vi "example_microFPGA.vi"() -> ()   [LabVIEW 2018]
panel:
  in  "write or read 2":u16(ring)=1 items=["read", "write"]
  out "Camera_sw_start_READ":u16(ring)=1 items=["Stop = 0", "Start = 1 "]
  in  "milliseconds to RUN":u32=2000
  out "value write confirm 11":bool=TRUE
  in  "Camera_sw_start_WRITE":u16(ring)=1 items=["Stop = 0", "Start = 1 "]
  out "camera_laser_delay_time_READ":u32(slide)=500 max=65535 step=1 scale=0.0..665535.0 scale format="%u us"
  out "value write confirm 10":bool=TRUE
  in  "camera_laser_delay_time_WRITE":u32(slide)=500 max=65535 step=1 scale=0.0..65535.0 scale format="%u us"
  out "camera_exposure_time_READ":u32(slide)=10000 max=65535 step=1 scale=0.0..1048575.0 scale format="%u us"
  out "value write confirm 9":bool=TRUE
  in  "camera_exposure_time_WRITE":u32(slide)=10000 max=1048580 step=1 scale=0.0..1048575.0 scale format="%u us"
  out "camera_readout_time_READ":u32(slide)=2000 max=65535 step=1 scale=0.0..665535.0 scale format="%u us"
  out "value write confirm 8":bool=TRUE
  in  "camera_readout_time_WRITE":u32(slide)=2000 max=65535 step=1 scale=0.0..65535.0 scale format="%u us"
  out "Camera_mode_READ":u16(ring)=1 items=["Passive = 0", "Active = 1 "]
  in  "Camera_mode_WRITE":u16(ring)=1 items=["Passive = 0", "Active = 1 "]
  out "value write confirm 7":bool=TRUE
  in  "camera_fire_pulse_time_WRITE":u32(slide)=1500 max=65535 step=1 scale=0.0..1048575.0 scale format="%u us"
  out "camera_fire_pulse_time_READ":u32(slide)=1500 max=65535 step=1 scale=0.0..1048575.0 scale format="%u us"
  in  "analog readout channel":u16(ring) items=["channel No 0", "channel No 1", "channel No 2", "channel No 3", "channel No 4", "channel No 5", "channel No 6", "channel No 7"]
  in  "laser channel":u16(ring)=1 items=["channel No 0", "channel No 1", "channel No 2", "channel No 3", "channel No 4", "channel No 5", "channel No 6", "channel No 7"]
  out "Servo_position_READ":u32(slide)=12706 max=65535 step=1 scale=0.0..65535.0 scale format="%u us"
  in  "Servo_channel":u16(ring) items=["channel No 0", "channel No 1", "channel No 2", "channel No 3", "channel No 4", "channel No 5", "channel No 6"]
  out "PWM_ratio_READ":u32(slide)=49 max=255 step=1 scale=0.0..255.0 scale format="%u us"
  in  "PWM_channel":u16(ring)=3 items=["channel No 0", "channel No 1", "channel No 2", "channel No 3", "channel No 4"]
  out "TTL_mode_READ":u16(ring)=1 items=["LO", "HIGH"]
  in  "TTL_channel":u16(ring)=3 items=["channel No 0", "channel No 1", "channel No 2", "channel No 3"]
  out "Laser_duration_READ":u32(slide)=9 max=65535 step=1 scale=0.0..65535.0 scale format="%u us"
  out "Laser_sequence_READ":bool[](array[boolean])=[FALSE, TRUE, FALSE, TRUE, FALSE, TRUE, FALSE, TRUE, FALSE, TRUE, FALSE, TRUE, FALSE, TRUE, FALSE, TRUE, FALSE, FALSE, FALSE, FALSE, FALSE, FALSE, FALSE, FALSE, FALSE, FALSE, FALSE, FALSE, FALSE, FALSE, FALSE, FALSE]
  out "Laser_mode_READ":u16(ring)=4 items=["OFF", "ON", "RISING", "FALLING", "FOLLOW"]
  out "value write confirm 6":bool=TRUE
  in  "write or read":u16(ring)=1 items=["read", "write"]
  out "analog value read (0 - 65535)":i32=6821
  out "value write confirm 5":bool
  out "value write confirm 4":bool
  out "value confirm":bool
  out "value write confirm 3":bool
  out "value write confirm 2":bool
  out "value write confirm":bool
  in  "Servo_position_WRITE":u32(slide)=12706 max=65535 step=1 scale=0.0..65535.0 scale format="%u us"
  out "Version":u16=3
  in  "PWM ratio":u32(slide)=49 max=255 step=1 scale=0.0..255.0 scale format="%u us"
  in  "TTL_channel_WRITE":u16(ring)=1 items=["LO", "HIGH"]
  in  "Laser_mode_WRITE":u16(ring)=4 items=["OFF", "ON", "RISING", "FALLING", "FOLLOW"]
  in  "Laser_sequence_WRITE":bool[](array[boolean])=[FALSE, TRUE, FALSE, TRUE, FALSE, TRUE, FALSE, TRUE, FALSE, TRUE, FALSE, TRUE, FALSE, TRUE, FALSE, TRUE]
  in  "Laser_duration_WRITE":u32(slide)=9 max=65535 step=1 scale=0.0..65535.0 scale format="%u us"
  in  "close Application":bool=TRUE
  in  "send parameters":bool
  # "analog input value read"
  # "initial readout of the MicroFPGA version after init"
  # "CAMERA"
  # "Laser / TTL / PWM / Servos"
  # "0"
  # "7"
  # "15"
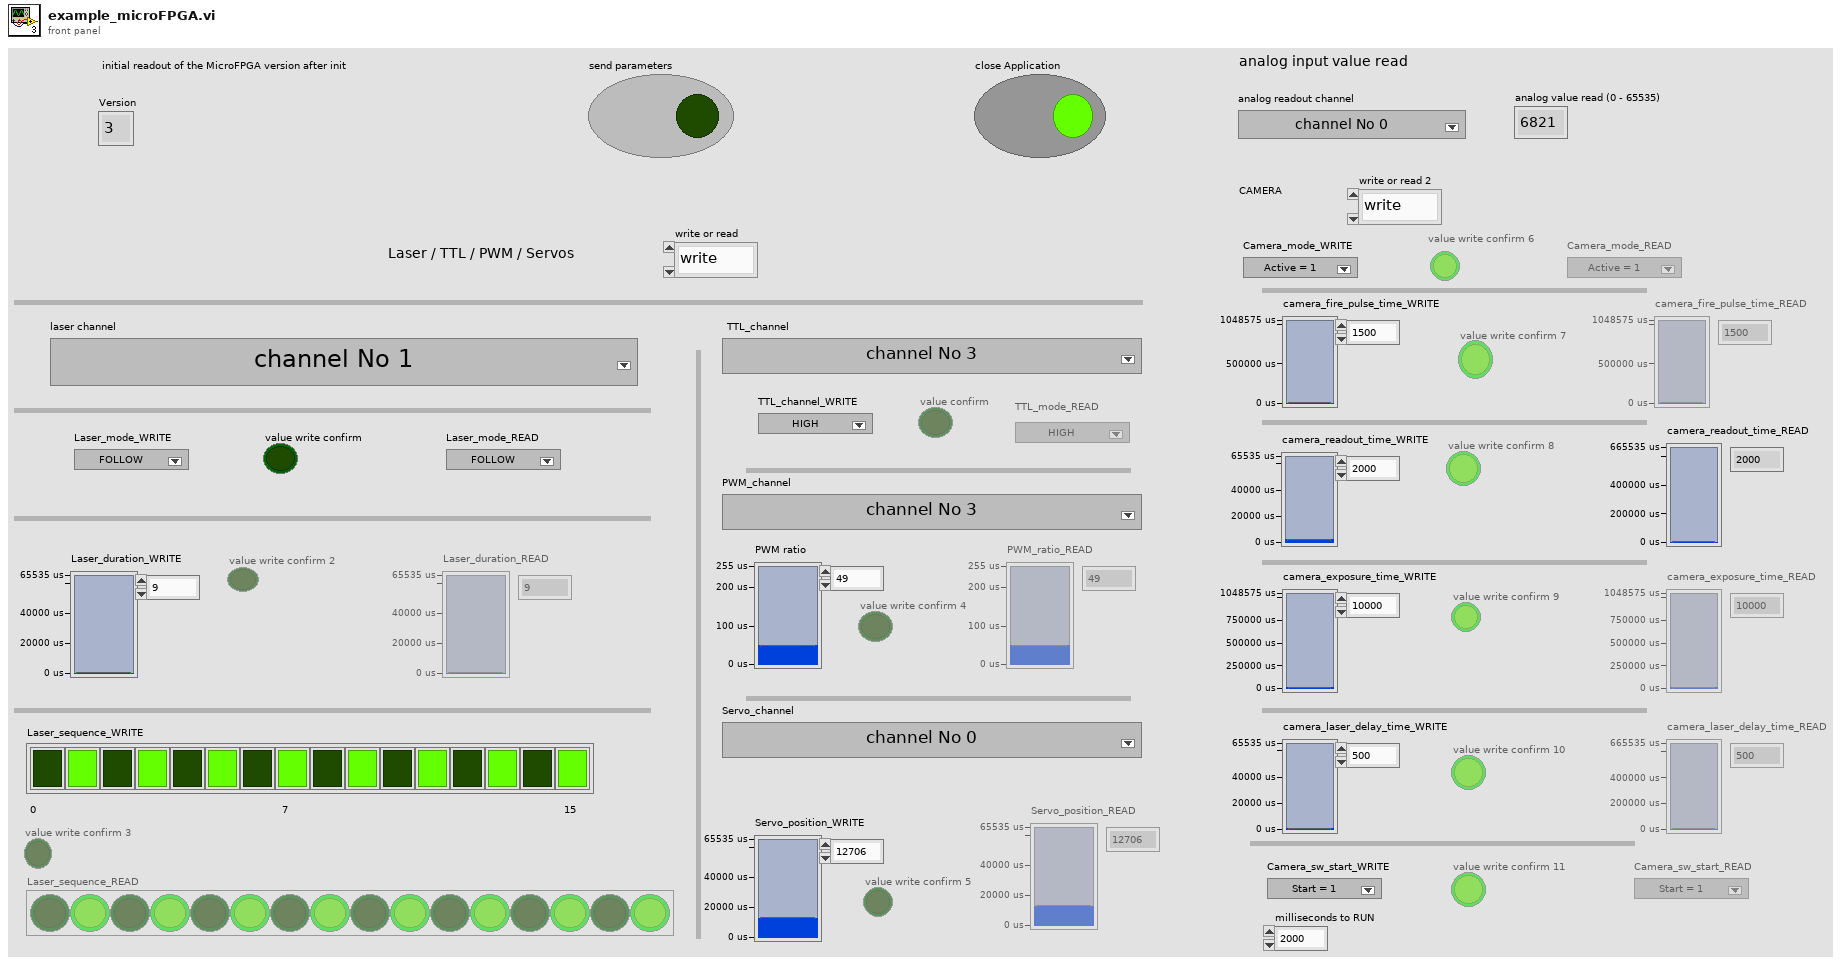
[diagram p1: front panel]
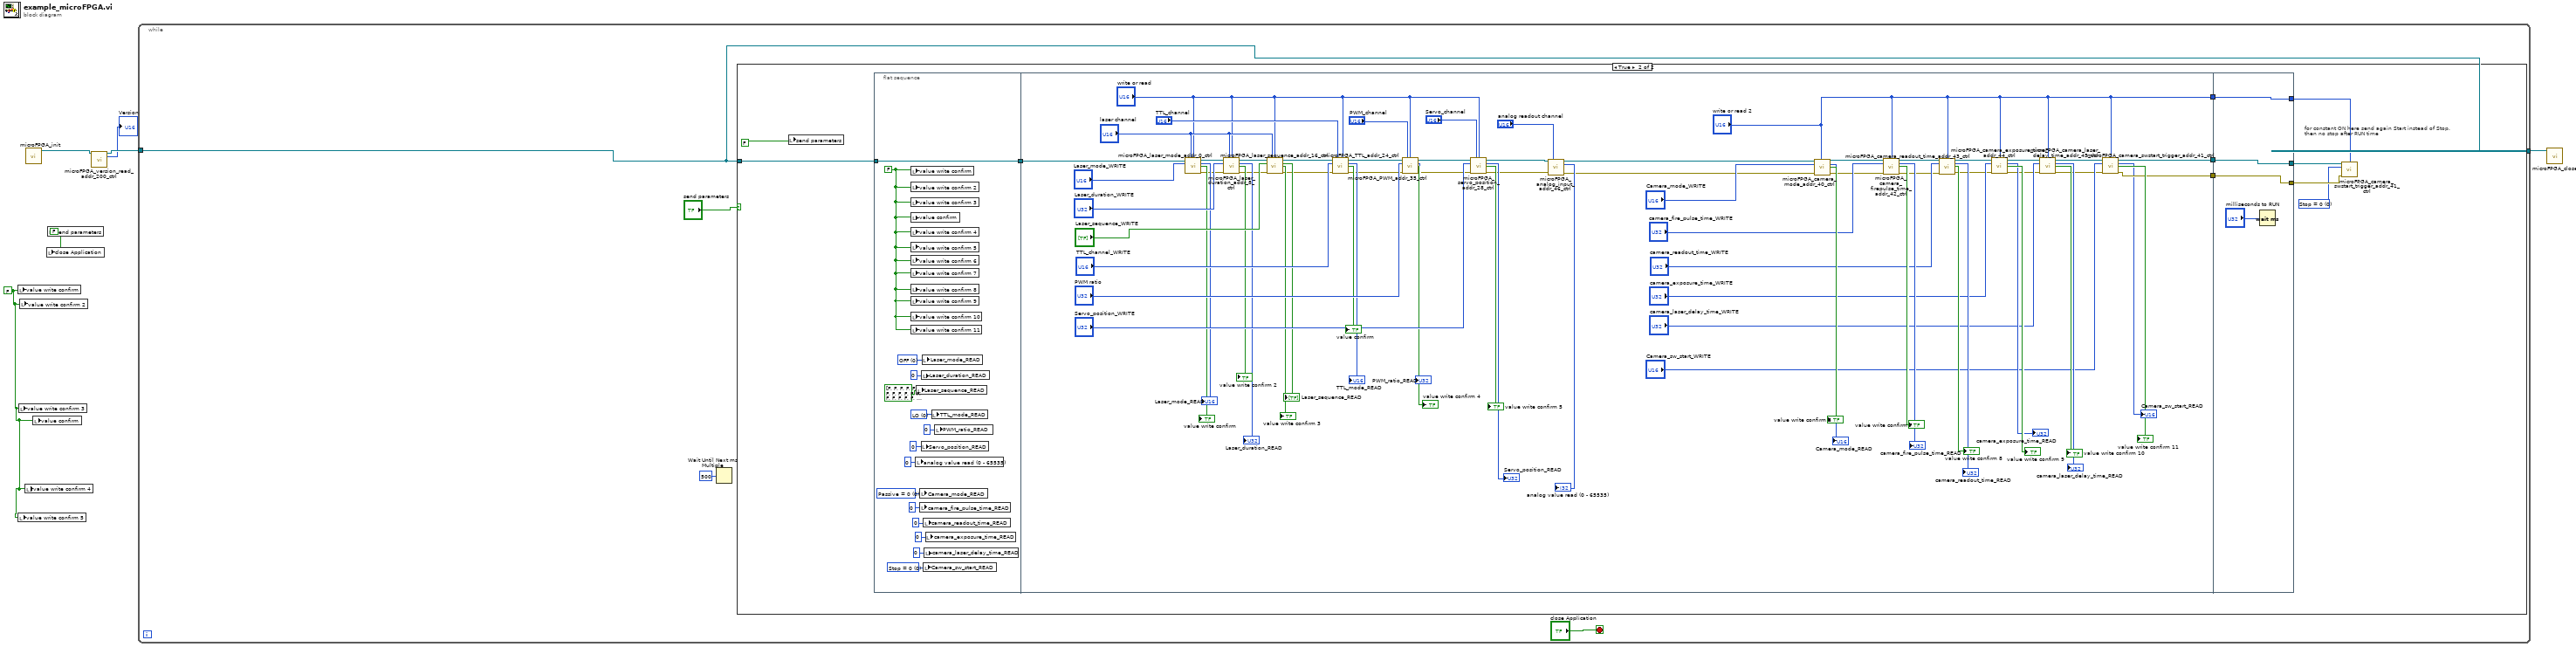
[diagram p0: block diagram]
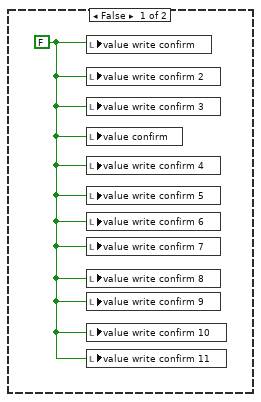
[diagram p2: hidden frame]
diagram:
  w1 = FALSE ("write")
  w6 = FALSE ("write")
  n1 = local write "value write confirm"(w1) -> ()
  n2 = local write "value write confirm 5"(w1) -> ()
  n3 = local write "value write confirm 3"(w1) -> ()
  n4 = local write "value write confirm 2"(w1) -> ()
  n5 = local write "value write confirm 4"(w1) -> ()
  n6 = call "microFPGA_init.vi"() -> ("VISA resource name out"=w4:refnum<visa-resource-name>)  [unwired: 10 in, 1 out]
  n7 = local write "value confirm"(w1) -> ()
  n8 = local write "close Application"(w6) -> ()
  n9 = local write "send parameters"(w6) -> ()
  n10 = call "microFPGA_version_read_addr_200_ctrl.vi"("VISA resource name"=w4) -> ("VISA resource name 2"=w3:refnum<visa-resource-name>, "Version"=→"Version":u16)  [unwired: 12 in, 1 out]
  n11 = while {
    tunnel: w3 -> [w7]
    tunnel: [w7] -> w5
    stop <- "close Application" stop-if-true
    n12 = Wait Until Next ms Multiple(millisecond multiple=u32 500) -> ()  [unwired: 1 out]
    n13 = case shown="True" "send parameters" {
      tunnel: w7 -> [_ w20]
      frame False {
        w11 = FALSE ("value write confirm")
        n14 = local write "value write confirm"(w11) -> ()
        n15 = local write "value write confirm 2"(w11) -> ()
        n16 = local write "value write confirm 3"(w11) -> ()
        n17 = local write "value confirm"(w11) -> ()
        n18 = local write "value write confirm 4"(w11) -> ()
        n19 = local write "value write confirm 5"(w11) -> ()
        n20 = local write "value write confirm 6"(w11) -> ()
        n21 = local write "value write confirm 7"(w11) -> ()
        n22 = local write "value write confirm 8"(w11) -> ()
        n23 = local write "value write confirm 9"(w11) -> ()
        n24 = local write "value write confirm 10"(w11) -> ()
        n25 = local write "value write confirm 11"(w11) -> ()
      }
      frame True {
        w12 = u16 0 items=["Stop = 0", "Start = 1 "] ("Camera_sw_start_WRITE 2")
        # "for constant ON here send again Start instead of Stop. \nthen no stop after RUN time"
        n26 = local write "send parameters"(FALSE ("write")) -> ()
        n27 = flat-sequence {
          tunnel: w20 -> [w36]
          tunnel: [w36] -> w13
          tunnel: [w53] -> w18
          tunnel: [w52] -> w17
          tunnel: ["write or read 2"] -> w15
          tunnel: w13 -> [w101]
          tunnel: [w110] -> w19
          tunnel: w18 -> [w110]
          tunnel: w17 -> [w109]
          tunnel: [w109] -> w16
          tunnel: w15 -> [w108]
          tunnel: [w108] -> w14
          frame #0 {
            w28 = u16 0 items=["Stop = 0", "Start = 1 "] ("Camera_sw_start_READ")
            w23 = u16 0 items=["Passive = 0", "Active = 1 "] ("Camera_mode_READ")
            w32 = u16 0 items=["LO", "HIGH"] ("TTL_mode_READ")
            w33 = u16 0 items=["OFF", "ON", "RISING", "FALLING", "CAMERA"] ("Laser_mode_READ")
            w22 = FALSE ("value write confirm")
            n28 = local write "value write confirm"(w22) -> ()
            n29 = local write "value write confirm 2"(w22) -> ()
            n30 = local write "value write confirm 3"(w22) -> ()
            n31 = local write "value confirm"(w22) -> ()
            n32 = local write "value write confirm 4"(w22) -> ()
            n33 = local write "value write confirm 5"(w22) -> ()
            n34 = local write "value write confirm 6"(w22) -> ()
            n35 = local write "value write confirm 7"(w22) -> ()
            n36 = local write "value write confirm 8"(w22) -> ()
            n37 = local write "value write confirm 9"(w22) -> ()
            n38 = local write "value write confirm 10"(w22) -> ()
            n39 = local write "value write confirm 11"(w22) -> ()
            n40 = local write "analog value read (0 - 65535)"(0 ("analog value read (0 - 65535)")) -> ()
            n41 = local write "Laser_sequence_READ"(bool[] [FALSE, FALSE, FALSE, FALSE, FALSE, FALSE, FALSE, FALSE, FALSE, FALSE, FALSE, FALSE, FALSE, FALSE, FALSE, FALSE, FALSE, FALSE, FALSE, FALSE, FALSE, FALSE, FALSE, FALSE, FALSE, FALSE, FALSE, FALSE, FALSE, FALSE, FALSE, FALSE] ("Laser_sequence_READ")) -> ()
            n42 = local write "Camera_mode_READ"(w23) -> ()
            n43 = local write "camera_fire_pulse_time_READ"(u32 0 ("camera_fire_pulse_time_READ")) -> ()
            n44 = local write "Servo_position_READ"(u32 0 ("Servo_position_READ")) -> ()
            n45 = local write "Laser_duration_READ"(u32 0 ("Laser_duration_READ")) -> ()
            n46 = local write "Laser_mode_READ"(w33) -> ()
            n47 = local write "Camera_sw_start_READ"(w28) -> ()
            n48 = local write "camera_readout_time_READ"(u32 0 ("camera_readout_time_READ")) -> ()
            n49 = local write "camera_laser_delay_time_READ"(u32 0 ("camera_laser_delay_time_READ")) -> ()
            n50 = local write "camera_exposure_time_READ"(u32 0 ("camera_exposure_time_READ")) -> ()
            n51 = local write "TTL_mode_READ"(w32) -> ()
            n52 = local write "PWM_ratio_READ"(u32 0 ("PWM_ratio_READ")) -> ()
          }
          frame #1 {
            n53 = call "microFPGA_laser_mode_addr_0_ctrl.vi"("VISA resource name"=w101, "laser channel"="laser channel", "write or read"="write or read", "Laser_mode_WRITE"="Laser_mode_WRITE") -> ("VISA resource name 2"=w99:refnum<visa-resource-name>, "Laser_mode_READ"=→"Laser_mode_READ":u16, "value write confirm"=→"value write confirm":bool, "error out"=w40:errorcluster)  [unwired: 7 in, 1 out]
            n54 = call "microFPGA_laser_duration_addr_8_ctrl.vi"("VISA resource name"=w99, "laser channel"="laser channel", "write or read"="write or read", "Laser_duration_WRITE"="Laser_duration_WRITE", "error in (no error)"=w40) -> ("VISA resource name 2"=w96:refnum<visa-resource-name>, "Laser_duration_READ"=→"Laser_duration_READ":u32, "value write confirm"=→"value write confirm 2":bool, "error out"=w41:errorcluster)  [unwired: 6 in, 1 out]
            n55 = call "microFPGA_laser_sequence_addr_16_ctrl.vi"("VISA resource name"=w96, "laser channel"="laser channel", "write or read"="write or read", "Laser_sequence_WRITE"="Laser_sequence_WRITE", "error in (no error)"=w41) -> ("VISA resource name 2"=w95:refnum<visa-resource-name>, "Laser_sequence_READ"=→"Laser_sequence_READ":bool[], "value write confirm"=→"value write confirm 3":bool, "error out"=w42:errorcluster)  [unwired: 6 in, 1 out]
            n56 = call "microFPGA_TTL_addr_24_ctrl.vi"("VISA resource name"=w95, "TTL_channel"="TTL_channel", "write or read"="write or read", "TTL_mode_WRITE"="TTL_channel_WRITE", "error in (no error)"=w42) -> ("VISA out"=w107:refnum<visa-resource-name>, "TTL_mode_READ"=→"TTL_mode_READ":u16, "value confirm"=→"value confirm":bool, "error out"=w43:errorcluster)  [unwired: 6 in, 1 out]
            n57 = call "microFPGA_PWM_addr_35_ctrl.vi"("VISA resource name"=w107, "PWM_channel"="PWM_channel", "write or read"="write or read", "PWM_ratio_WRITE"="PWM ratio", "error in (no error)"=w43) -> ("VISA resource name 2"=w104:refnum<visa-resource-name>, "PWM_ratio_READ"=→"PWM_ratio_READ":u32, "value write confirm"=→"value write confirm 4":bool, "error out"=w44:errorcluster)  [unwired: 6 in, 1 out]
            n58 = call "microFPGA_servo_position_addr_28_ctrl.vi"("VISA resource name"=w104, "Servo_channel"="Servo_channel", "write or read"="write or read", "Servo_position_WRITE"="Servo_position_WRITE", "error in (no error)"=w44) -> ("VISA resource name 2"=w103:refnum<visa-resource-name>, "Servo_position_READ"=→"Servo_position_READ":u32, "value write confirm"=→"value write confirm 5":bool, "error out"=w45:errorcluster)  [unwired: 6 in, 1 out]
            n59 = call "microFPGA_analog_input_addr_46_ctrl.vi"("VISA resource name"=w103, "analog readout channel"="analog readout channel", "error in (no error)"=w45) -> ("VISA resource name 2"=w87:refnum<visa-resource-name>, "analog value read"=→"analog value read (0 - 65535)":i32, "error out"=w46:errorcluster)  [unwired: 9 in, 1 out]
            n60 = call "microFPGA_camera_mode_addr_40_ctrl.vi"("VISA resource name"=w87, "write or read"="write or read 2", "Camera_mode_WRITE"="Camera_mode_WRITE", "error in (no error)"=w46) -> ("VISA resource name 2"=w74:refnum<visa-resource-name>, "Camera_mode_READ"=→"Camera_mode_READ":u16, "value write confirm"=→"value write confirm 6":bool, "error out"=w47:errorcluster)  [unwired: 7 in, 1 out]
            n61 = call "microFPGA_camera_firepulse_time_addr_42_ctrl.vi"("VISA resource name"=w74, "write or read"="write or read 2", "camera_fire_pulse_time_WRITE"="camera_fire_pulse_time_WRITE", "error in (no error)"=w47) -> ("VISA resource name 2"=w65:refnum<visa-resource-name>, "camera_fire_pulse_time_READ"=→"camera_fire_pulse_time_READ":u32, "value write confirm"=→"value write confirm 7":bool, "error out"=w48:errorcluster)  [unwired: 7 in, 1 out]
            n62 = call "microFPGA_camera_readout_time_addr_43_ctrl.vi"("VISA resource name"=w65, "write or read"="write or read 2", "camera_readout_time_WRITE"="camera_readout_time_WRITE", "error in (no error)"=w48) -> ("VISA resource name 2"=w63:refnum<visa-resource-name>, "camera_readout_time_READ"=→"camera_readout_time_READ":u32, "value write confirm"=→"value write confirm 8":bool, "error out"=w49:errorcluster)  [unwired: 7 in, 1 out]
            n63 = call "microFPGA_camera_exposure_time_addr_44_ctrl.vi"("VISA resource name"=w63, "write or read"="write or read 2", "camera_exposure_time_WRITE"="camera_exposure_time_WRITE", "error in (no error)"=w49) -> ("VISA resource name 2"=w62:refnum<visa-resource-name>, "camera_exposure_time_READ"=→"camera_exposure_time_READ":u32, "value write confirm"=→"value write confirm 9":bool, "error out"=w50:errorcluster)  [unwired: 7 in, 1 out]
            n64 = call "microFPGA_camera_laser_delay_time_addr_45_ctrl.vi"("VISA resource name"=w62, "write or read"="write or read 2", "camera_laser_delay_time_WRITE"="camera_laser_delay_time_WRITE", "error in (no error)"=w50) -> ("VISA resource name 2"=w56:refnum<visa-resource-name>, "camera_laser_delay_time_READ"=→"camera_laser_delay_time_READ":u32, "value write confirm"=→"value write confirm 10":bool, "error out"=w51:errorcluster)  [unwired: 7 in, 1 out]
            n65 = call "microFPGA_camera_swstart_trigger_addr_41_ctrl.vi"("VISA resource name"=w56, "write or read"="write or read 2", "Camera_sw_start_WRITE"="Camera_sw_start_WRITE", "error in (no error)"=w51) -> ("VISA resource name 2"=w53:refnum<visa-resource-name>, "Camera_sw_start_READ"=→"Camera_sw_start_READ":u16, "value write confirm"=→"value write confirm 11":bool, "error out"=w52:errorcluster)  [unwired: 7 in, 1 out]
          }
          frame #2 {
            n66 = Wait (ms)(milliseconds to wait="milliseconds to RUN") -> ()  [unwired: 1 out]
          }
        }
        n67 = call "microFPGA_camera_swstart_trigger_addr_41_ctrl.vi"("VISA resource name"=w19, "write or read"=w14, "Camera_sw_start_WRITE"=w12, "error in (no error)"=w16) -> ()  [unwired: 7 in, 5 out]
      }
    }
  }
  n68 = call "microFPGA_close.vi"("VISA resource name"=w5) -> ()  [unwired: 11 in]
